vi "HashingVectorizer.vi"(8 "error in":errorcluster caption="entrée d'erreur", 11 "HashingVectorizer":T1={"encoding"="utf-8", "decode_error"="strict", "strip_accents"="None", "lowercase"=TRUE, "preprocessor"="None", "tokenizer"="None", "stop_words"={"Type"="None", "list"=[]}, "token_pattern"="(?u)\\b\\w\\w+\\b", "ngram_range"={"min_n"=1, "max_n"=1}, "analyzer"="word", "n_features"=1048576, "binary"=FALSE, "norm"="l2", "alternate_sign"=TRUE, "dtype"="float"}) -> (0 "error out":errorcluster caption="sortie d'erreur", 3 "HashingVectorizer.lvclass":refnum<class "HashingVectorizer.lvclass">)   [LabVIEW 2020]
doc: "Convert a collection of text documents to a matrix of token occurrences\n\nIt turns a collection of text documents into a scipy.sparse matrix holding token occurrence counts (or binary occurrence information), possibly normalized as token frequencies if norm=’l1’ or projected on the euclidean unit sphere if norm=’l2’.\n\nThis text vectorizer implementation uses the hashing trick to find the token string name to feature integer index mapping.\n\nThis strategy has several advantages :\n\n- it is very low memory scalable to large datasets as there is no need to store a vocabulary dictionary in memory\n\n- it is fast to pickle and un-pickle as it holds no state besides the constructor parameters\n\n- it can be used in a streaming (partial fit) or parallel pipeline as there is no state computed during fit.\n\nThere are also a couple of cons (vs using a CountVectorizer with an in-memory vocabulary) :\n\n- there is no way to compute the inverse transform (from feature indices to string feature names) which can be a problem when trying to introspect which features are most important to a model.\n\n- there can be collisions: distinct tokens can be mapped to the same feature index. However in practice this is rarely an issue if n_features is large enough (e.g. 2 ** 18 for text classification problems).\n\n- no IDF weighting as this would render the transformer stateful.\n\n\nParameters : \n\n- encoding : string, default=’utf-8’\nIf bytes or files are given to analyze, this encoding is used to decode.\n\n- decode_error : {‘strict’, ‘ignore’, ‘replace’}, default=’strict’\nInstruction on what to do if a byte sequence is given to analyze that contains characters not of the given encoding. By default, it is ‘strict’, meaning that a UnicodeDecodeError will be raised. Other values are ‘ignore’ and ‘replace’.\n\n- strip_accents : {‘ascii’, ‘unicode’}, default=None\nRemove accents and perform other character normalization during the preprocessing step. ‘ascii’ is a fast method that only works on characters that have an direct ASCII mapping. ‘unicode’ is a slightly slower method that works on any characters. None (default) does nothing.\n\n- lowercase : bool, default=True\nConvert all characters to lowercase before tokenizing.\n\n- preprocessor : callable, default=None\nOverride the preprocessing (string transformation) stage while preserving the tokenizing and n-grams generation steps. Only applies if analyzer is not callable.\n\n- tokenizer : callable, default=None\nOverride the string tokenization step while preserving the preprocessing and n-grams generation steps. Only applies if analyzer == 'word'.\n\n- stop_words : string {‘english’}, list, default=None\nIf ‘english’, a built-in stop word list for English is used. There are several known issues with ‘english’ and you should consider an alternative (see Using stop words).\n\nIf a list, that list is assumed to contain stop words, all of which will be removed from the resulting tokens. Only applies if analyzer == 'word'.\n\n- token_pattern : string\nRegular expression denoting what constitutes a “token”, only used if analyzer == 'word'. The default regexp selects tokens of 2 or more alphanumeric characters (punctuation is completely ignored and always treated as a token separator).\n\n- ngram_range : tuple (min_n, max_n), default=(1, 1)\nThe lower and upper boundary of the range of n-values for different n-grams to be extracted. All values of n such that min_n <= n <= max_n will be used. For example an ngram_range of (1, 1) means only unigrams, (1, 2) means unigrams and bigrams, and (2, 2) means only bigrams. Only applies if analyzer is not callable.\n\n- analyzer : string, {‘word’, ‘char’, ‘char_wb’} or callable, default=’word’\nWhether the feature should be made of word or character n-grams. Option ‘char_wb’ creates character n-grams only from text inside word boundaries; n-grams at the edges of words are padded with space.\n\nIf a callable is passed it is used to extract the sequence of features out of the raw, unprocessed input.\n\n- n_features : int, default=(2 ** 20)\nThe number of features (columns) in the output matrices. Small numbers of features are likely to cause hash collisions, but large numbers will cause larger coefficient dimensions in linear learners.\n\n- binary : bool, default=False.\nIf True, all non zero counts are set to 1. This is useful for discrete probabilistic models that model binary events rather than integer counts.\n\n- norm : {‘l1’, ‘l2’}, default=’l2’\nNorm used to normalize term vectors. None for no normalization.\n\n- alternate_sign : bool, default=True\nWhen True, an alternating sign is added to the features as to approximately conserve the inner product in the hashed space even for small n_features. This approach is similar to sparse random projection.\n\n- dtype : type, default=np.float64\nType of the matrix returned by fit_transform() or transform().\n\n\n\nMethods : \n\n- Decode : Decode the input into a string of unicode symbols. The decoding strategy depends on the vectorizer parameters.\n\nParameters : doc : str\n The string to decode.\n\nReturns : doc : str\n A string of unicode symbols.\n\n\n- Fit : Does nothing: this transformer is stateless.\n\nParameters : X : ndarray of shape [n_samples, n_features]\n Training data.\n\n- Fit Transform : Transform a sequence of documents to a document-term matrix.\n\nParameters : X : iterable over raw text documents, length = n_samples\nSamples. Each sample must be a text document (either bytes or unicode strings, file name or file object depending on the constructor argument) which will be tokenized and hashed.\n\nReturns : X : sparse matrix of shape (n_samples, n_features)\n Document-term matrix.\n\n- Transform : Transform a sequence of documents to a document-term matrix.\n\nParameters : X : iterable over raw text documents, length = n_samples\nSamples. Each sample must be a text document (either bytes or unicode strings, file name or file object depending on the constructor argument) which will be tokenized and hashed.\n\nReturns : X : sparse matrix of shape (n_samples, n_features)\n Document-term matrix."
uses:
  HashingVectorizer.lvclass
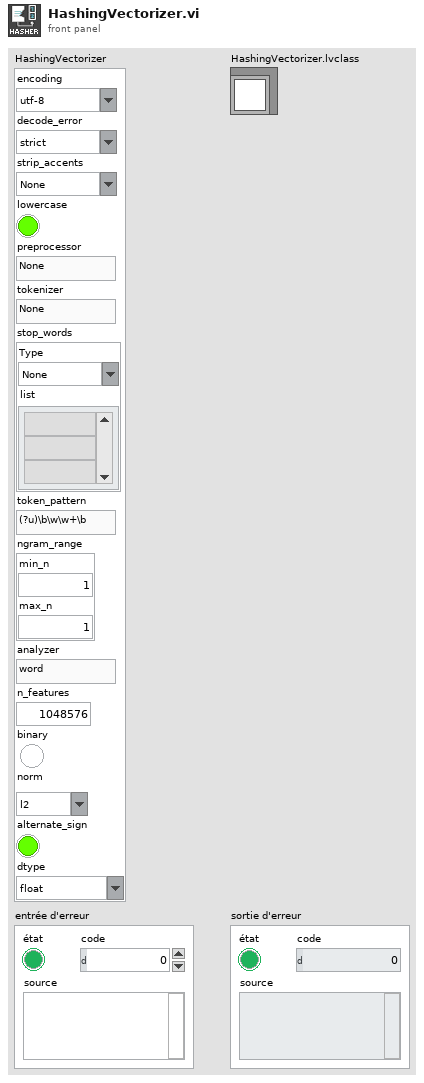
[diagram p1: front panel]
types:
  T1 = cluster{"encoding":string, "decode_error":string, "strip_accents":string, "lowercase":bool, "preprocessor":string, "tokenizer":string, "stop_words":cluster{"Type":string, "list":string[]}, "token_pattern":string, "ngram_range":cluster{"min_n":i32, "max_n":i32}, "analyzer":string, "n_features":i32, "binary":bool, "norm":string, "alternate_sign":bool, "dtype":string}
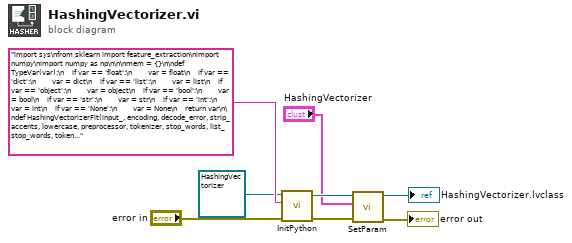
[diagram p0: block diagram]
diagram:
  n1 = call-dynamic "InitPython.vi"("error in (no error)"="error in", "Python Instruction"="import sys\nfrom sklearn import feature_extraction\nimport numpy\nimport numpy as np\n\n\nmem = {}\n\ndef TypeVar(var):\n    if var == 'float':\n        var = float\n    if var == 'dict':\n        var = dict\n    if var == 'list':\n        var = list\n    if var == 'object':\n        var = object\n    if var == 'bool':\n        var = bool\n    if var == 'str':\n        var = str\n    if var == 'int':\n        var = int\n    if var == 'None':\n        var = None\n    return var\n\ndef HashingVectorizerFit(input_, encoding, decode_error, strip_accents, lowercase, preprocessor, tokenizer, stop_words, list_stop_words, token_pattern, min_n, max_n, analyzer, n_features, binary, norm, alternate_sign, dtype, X, doc):\n    X = eval(X)\n    dtype = TypeVar(dtype)\n    list_analyzer = ['word', 'char', 'char_wb']\n    if tokenizer == 'None' or tokenizer == '':\n        tokenizer = None\n    else:\n        tokenizer = eval(tokenizer)\n    if preprocessor == 'None' or preprocessor == '':\n        preprocessor = None\n    else:\n        preprocessor = eval(preprocessor)\n    if strip_accents == 'None':\n        strip_accents = None\n    if stop_words == 'None':\n        stop_words = None\n    elif stop_words == 'list':\n        stop_words = list_stop_words\n    else: \n        pass\n    if analyzer not in list_analyzer:\n        analyzer = eval(analyzer) \n    try:\n        HashingVectorizer = feature_extraction.text.HashingVectorizer(input_, encoding, decode_error, strip_accents, lowercase, preprocessor, tokenizer, stop_words, token_pattern, (min_n, max_n), analyzer, n_features, binary, norm, alternate_sign, dtype).fit(X)\n        mem['FitHashingVectorizer'] = HashingVectorizer\n        return str('OK')\n    except:\n        erreur = sys.exc_info()\n        typerr = u\"%s\" % (erreur[0])\n        typerr = typerr[typerr.find(\"'\")+1:typerr.rfind(\"'\")]\n        msgerr = u\"%s\" % (erreur[1])\n        message = str('/!\\\\ {0} : {1}'. format(typerr,msgerr))\n        return message \n\ndef HashingVectorizerFitTransform(input_, encoding, decode_error, strip_accents, lowercase, preprocessor, tokenizer, stop_words, list_stop_words, token_pattern, min_n, max_n, analyzer, n_features, binary, norm, alternate_sign, dtype, X, doc):\n    X = eval(X)\n    dtype = TypeVar(dtype)\n    list_analyzer = ['word', 'char', 'char_wb']\n    if tokenizer == 'None' or tokenizer == '':\n        tokenizer = None\n    else:\n        tokenizer = eval(tokenizer)\n    if preprocessor == 'None' or preprocessor == '':\n        preprocessor = None\n    else:\n        preprocessor = eval(preprocessor)\n    if strip_accents == 'None':\n        strip_accents = None\n    if stop_words == 'None':\n        stop_words = None\n    elif stop_words == 'list':\n        stop_words = list_stop_words\n    else: \n        pass\n    if analyzer not in list_analyzer:\n        analyzer = eval(analyzer) \n    try:\n        HashingVectorizer = feature_extraction.text.HashingVectorizer(input_, encoding, decode_error, strip_accents, lowercase, preprocessor, tokenizer, stop_words, token_pattern, (min_n, max_n), analyzer, n_features, binary, norm, alternate_sign, dtype).fit_transform(X)\n        Mat = HashingVectorizer.tocoo()\n        return str(list(zip(Mat.row, Mat.col, Mat.data)))\n    except:\n        erreur = sys.exc_info()\n        typerr = u\"%s\" % (erreur[0])\n        typerr = typerr[typerr.find(\"'\")+1:typerr.rfind(\"'\")]\n        msgerr = u\"%s\" % (erreur[1])\n        message = str('/!\\\\ {0} : {1}'. format(typerr,msgerr))\n        return message \n    \ndef HashingVectorizerTransform(input_, encoding, decode_error, strip_accents, lowercase, preprocessor, tokenizer, stop_words, list_stop_words, token_pattern, min_n, max_n, analyzer, n_features, binary, norm, alternate_sign, dtype, X, doc):\n    X = eval(X)\n    dtype = TypeVar(dtype)\n    list_analyzer = ['word', 'char', 'char_wb']\n    if tokenizer == 'None' or tokenizer == '':\n        tokenizer = None\n    else:\n        tokenizer = eval(tokenizer)\n    if preprocessor == 'None' or preprocessor == '':\n        preprocessor = None\n    else:\n        preprocessor = eval(preprocessor)\n    if strip_accents == 'None':\n        strip_accents = None\n    if stop_words == 'None':\n        stop_words = None\n    elif stop_words == 'list':\n        stop_words = list_stop_words\n    else: \n        pass\n    if analyzer not in list_analyzer:\n        analyzer = eval(analyzer) \n    try:\n        HashingVectorizer = mem['FitHashingVectorizer'].transform(X)\n        Mat = HashingVectorizer.tocoo()\n        return str(list(zip(Mat.row, Mat.col, Mat.data)))\n    except:\n        erreur = sys.exc_info()\n        typerr = u\"%s\" % (erreur[0])\n        typerr = typerr[typerr.find(\"'\")+1:typerr.rfind(\"'\")]\n        msgerr = u\"%s\" % (erreur[1])\n        message = str('/!\\\\ {0} : {1}'. format(typerr,msgerr))\n        return message\n    \ndef HashingVectorizerDecode(input_, encoding, decode_error, strip_accents, lowercase, preprocessor, tokenizer, stop_words, list_stop_words, token_pattern, min_n, max_n, analyzer, n_features, binary, norm, alternate_sign, dtype, X, doc):\n    X = eval(X)\n    dtype = TypeVar(dtype)\n    list_analyzer = ['word', 'char', 'char_wb']\n    if tokenizer == 'None' or tokenizer == '':\n        tokenizer = None\n    else:\n        tokenizer = eval(tokenizer)\n    if preprocessor == 'None' or preprocessor == '':\n        preprocessor = None\n    else:\n        preprocessor = eval(preprocessor)\n    if strip_accents == 'None':\n        strip_accents = None\n    if stop_words == 'None':\n        stop_words = None\n    elif stop_words == 'list':\n        stop_words = list_stop_words\n    else: \n        pass\n    if analyzer not in list_analyzer:\n        analyzer = eval(analyzer) \n    try:\n        HashingVectorizer = feature_extraction.text.HashingVectorizer(input_, encoding, decode_error, strip_accents, lowercase, preprocessor, tokenizer, stop_words, token_pattern, (min_n, max_n), analyzer, n_features, binary, norm, alternate_sign, dtype).decode(doc)\n        return str(HashingVectorizer)\n    except:\n        erreur = sys.exc_info()\n        typerr = u\"%s\" % (erreur[0])\n        typerr = typerr[typerr.find(\"'\")+1:typerr.rfind(\"'\")]\n        msgerr = u\"%s\" % (erreur[1])\n        message = str('/!\\\\ {0} : {1}'. format(typerr,msgerr))\n        return message", "Scikit-learn en entrée"=refnum<class "HashingVectorizer.lvclass"> refnum ("HashingVectorizer.lvclass")) -> ("error out"=w4:errorcluster, "Scikit-learn en sortie"=w5:refnum<class "HashingVectorizer.lvclass">)  [unwired: 7 in]
  n2 = call-dynamic "SetParam.vi"("error in (no error)"=w4, "HashingVectorizer"="HashingVectorizer", "HashingVectorizer.lvclass"=w5) -> ("error out"=→"error out":errorcluster, "HashingVectorizer.lvclass"=→"HashingVectorizer.lvclass":refnum<class "HashingVectorizer.lvclass">)  [unwired: 7 in]
